vi "Test_WriteItemTwice_VariantType_Replaced.vi"(8 "error in (no error)":errorcluster, 11 "TestCase in":refnum<class "TestComposedLookupTable.lvclass">) -> (0 "error out":errorcluster, 3 "TestCase out":refnum<class "TestComposedLookupTable.lvclass">)   [LabVIEW 2017, in "TestComposedLookupTable.lvclass"]
uses:
  TestComposedLookupTable.lvclass
  Source/LookupTable/LookupTable.lvclass/LookupTable.ctl
  795aeb50-7324-4620-a4ed-731e649c4fc8.vi
  0f4fd84d-09cb-4032-bd40-49a8e65684c7.vi
  Source/LookupTable/Read Table Reference.vi
  795aeb50-7324-4620-a4ed-731e649c4fc8.vi/555e17fd-c62d-4de3-9e72-28cd8cd95cf1.vi
  0f4fd84d-09cb-4032-bd40-49a8e65684c7.vi/116419bb-ca81-4b97-97e3-fadb8f39adaa.vi
  Source/LookupTable/LookupTable.lvclass
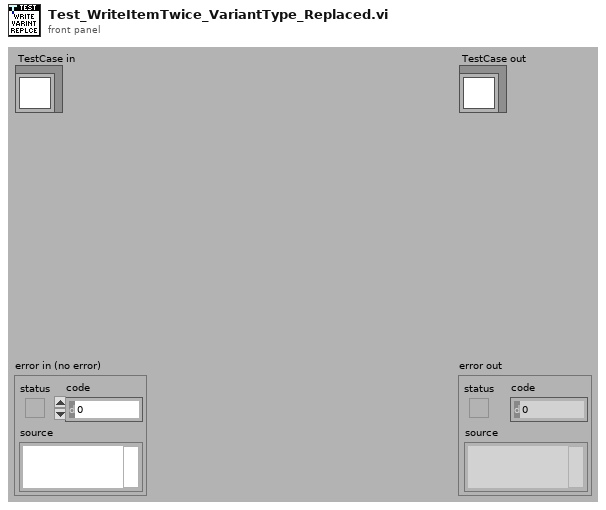
[diagram p1: front panel]
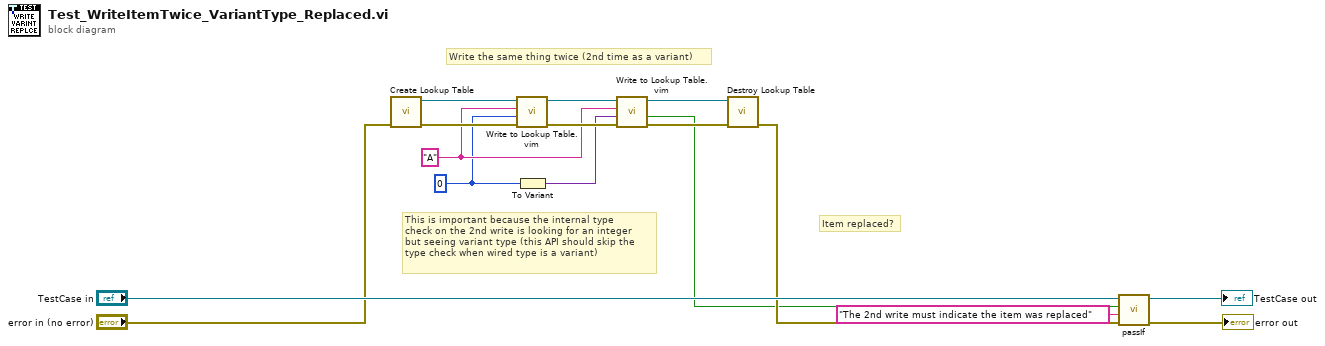
[diagram p0: block diagram]
diagram:
  w1 = 0
  w10 = "A" ("Item Name")
  # "This is important because the internal type\ncheck on the 2nd write is looking for an integer\nbut seeing variant type (this API should skip the\ntype check when wired type is a variant)"
  # "Write the same thing twice (2nd time as a variant)"
  # "Item replaced?"
  n1 = call "Create Lookup Table.vi"("error in (no error)"="error in (no error)") -> ("error out"=w16:errorcluster, "LookupTable Reference"=w8:refnum<data-value>)  [unwired: 9 in]
  n2 = call "Write to Lookup Table.vim"("error in (no error)"=w16, "Item"=w1, "Item Name"=w10, "LookupTable Reference"=w8) -> ("error out"=w11:errorcluster, "LookupTable Reference Out"=w12:refnum<data-value>)  [unwired: 5 in, 1 out]
  n3 = To Variant(anything=w1) -> (Variant=w2:variant)
  n4 = call "Write to Lookup Table.vim"("error in (no error)"=w11, "Item"=w2, "Item Name"=w10, "LookupTable Reference"=w12) -> ("error out"=w5:errorcluster, "Replaced?"=w3:bool, "LookupTable Reference Out"=w6:refnum<data-value>)  [unwired: 5 in]
  n5 = call "Destroy Lookup Table.vi"("error in (no error)"=w5, "LookupTable Reference"=w6) -> ("error out"=w4:errorcluster)  [unwired: 9 in]
  n6 = call-dynamic "passIf.vi"("error in (no error)"=w4, "message (\"\")"="The 2nd write must indicate the item was replaced" ("message (\"\")"), "pass"=w3, "TestCase in"="TestCase in") -> ("error out"=→"error out":errorcluster, "TestCase out"=→"TestCase out":refnum<class "TestComposedLookupTable.lvclass">)  [unwired: 6 in]
